vi "Sub_neighboring_pin_locations.vi"(9 "Setup Parameters":T1, 10 "FEA Nodes":i32[](array[numeric]), 11 "Initial Pin Location":i32) -> (1 "Unique Samples":i32[](array[numeric]))   [LabVIEW 2019]
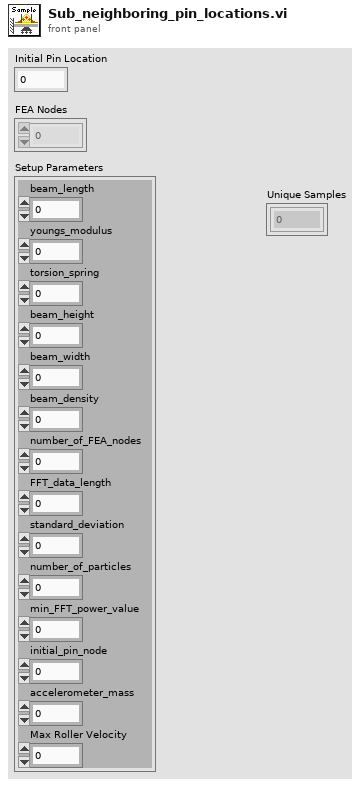
[diagram p1: front panel]
types:
  T1 = cluster{"beam_length":dbl, "youngs_modulus":dbl, "torsion_spring":dbl, "beam_height":dbl, "beam_width":dbl, "beam_density":dbl, "number_of_FEA_nodes":i32, "FFT_data_length":i32, "standard_deviation":dbl, "number_of_particles":i32, "min_FFT_power_value":dbl, "initial_pin_node":i32, "accelerometer_mass":dbl, "Max Roller Velocity":dbl}
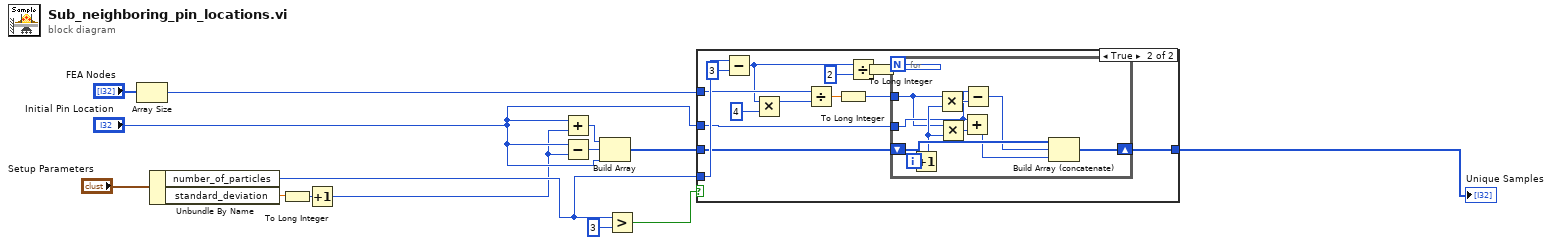
[diagram p0: block diagram]
diagram:
  n1 = Array Size(array="FEA Nodes") -> (size(s)=w4:i32)
  n2 = Unbundle By Name("Setup Parameters") -> ("number_of_particles"=w9:i32, "standard_deviation"=w3:dbl)
  n3 = To Long Integer(number=w3) -> (32bit integer=w2:i32)
  n4 = Increment(x=w2) -> (x+1=w1:i32)
  n5 = Add(x="Initial Pin Location", y=w1) -> (x+y=w12:i32)
  n6 = Subtract(x="Initial Pin Location", y=w1) -> (x-y=w13:i32)
  n7 = Build Array(w12, w13, "Initial Pin Location") -> (w8:i32[])
  n8 = Greater?(x=w9, y=3) -> (0:w10:bool)
  n9 = case shown="True" w10 {
    tunnel: w9 -> [_ w29]
    tunnel: w4 -> [_ w27]
    tunnel: w8 -> [w15 w19]
    tunnel: [w15 w17] -> w7
    tunnel: "Initial Pin Location" -> [_ w18]
    frame False {
    }
    frame True {
      n10 = Subtract(x=w29, y=3) -> (x-y=w26:i32)
      n11 = Multiply(x=w26, y=4) -> (x*y=w25:i32)
      n12 = Divide(x=w27, y=w25) -> (x/y=w20:dbl)
      n13 = To Long Integer(number=w20) -> (32bit integer=w16:i32)
      n14 = Divide(x=w26, y=2) -> (x/y=w23:dbl)
      n15 = To Long Integer(number=w23) -> (32bit integer=w21:i32)
      n16 = for {
        N: w21 -> [_]
        tunnel: w16 -> [w30]
        tunnel: w18 -> [w31]
        shift-right: [w38] -> w17
        shift-left: w19 -> [w39]
        i -> [w33]
        n17 = Increment(x=w33) -> (x+1=w32:i32)
        n18 = Multiply(x=w30, y=w32) -> (x*y=w35:i32)
        n19 = Multiply(x=w30, y=w32) -> (x*y=w34:i32)
        n20 = Add(x=w31, y=w34) -> (x+y=w37:i32)
        n21 = Subtract(x=w31, y=w35) -> (x-y=w36:i32)
        n22 = Build Array (concatenate)(w39, w36, w37) -> (w38:i32[])
      }
    }
  }
  "Unique Samples" <- w7
